vi "frontp_write_subpanel_refrerences.vi"(8 "error in (no error)":errorcluster, 10 "GUI_subpanels":T1, 11 "front_panel in":refnum<class "front_panel.lvclass">) -> (0 "error out":errorcluster, 3 "front_panel out":refnum<class "front_panel.lvclass">)   [LabVIEW 2015, in "front_panel.lvclass"]
uses:
  front_panel.lvclass
  gui_subpanel_references.ctl
  front_panel.lvclass/front_panel.ctl
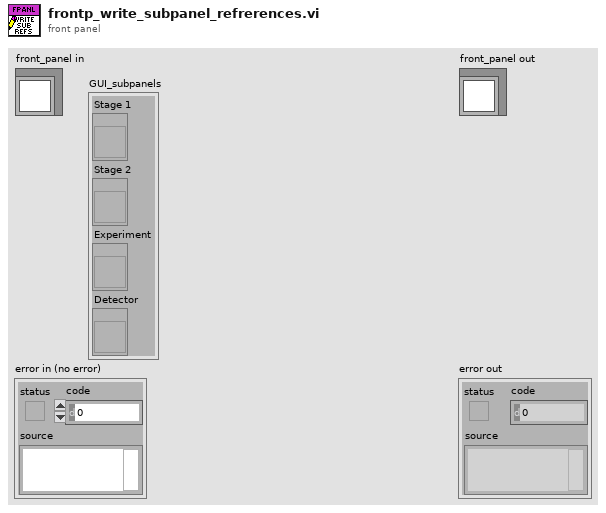
[diagram p1: front panel]
types:
  T1 = typedef "gui_subpanel_references.ctl" = cluster{"Stage 1":refnum<vi>, "Stage 2":refnum<vi>, "Experiment":refnum<vi>, "Detector":refnum<vi>}
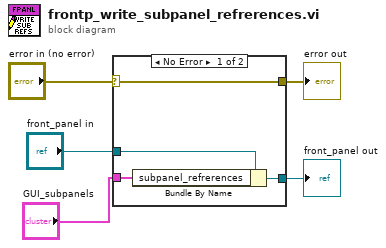
[diagram p0: block diagram]
diagram:
  n1 = case shown="No Error" "error in (no error)" {
    selector: "error in (no error)" -> [w9 w10]
    tunnel: [w9 w10] -> w4
    tunnel: [w7 w11] -> w2
    tunnel: "front_panel in" -> [w8 w11]
    tunnel: "GUI_subpanels" -> [w6 _]
    frame No Error {
      n2 = Bundle By Name(cluster=w8, "subpanel_refrerences"=w6) -> (w7:refnum<class "front_panel.lvclass">)
    }
    frame Error {
    }
  }
  "error out" <- w4
  "front_panel out" <- w2
